vi "ctet_dmm_User Main.vi"() -> ()   [LabVIEW 2019, in "ctet_dmm User Library.lvlib"]
uses:
  ctet_dmm User Library.lvlib
  Servers/ctet_dmm/ctet_dmm Class/typeDefs/Server State Data.ctl
  Types/ctet_dmm.ctl
  Servers/ctet_dmm/ctet_dmm Class/RPC Messages/measurementservice_DMMConfigResponse/measurementservice_DMMConfigResponse_Data.ctl
  Servers/ctet_dmm/ctet_dmm Class/RPC Messages/measurementservice_ErrorOut/measurementservice_ErrorOut_Data.ctl
  Servers/ctet_dmm/ctet_dmm Class/ctet_dmm.lvclass/ctet_dmm.ctl
  Servers/ctet_dmm/ctet_dmm Class/ctet_dmm.lvclass
panel:
  in  "Stop":bool
  in  "Server Address":string="0.0.0.0:50051"
  in  "Server Certificate File (.crt)":path
  in  "Server Key File (.key)":path
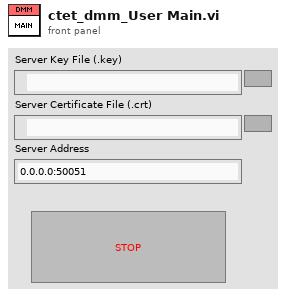
[diagram p1: front panel]
types:
  T1 = typedef "ctet_dmm User Library.lvlib/ctet_dmm.ctl" = cluster{"DMMSession":refnum<k15>, "measurementservice_DMMConfigResponse_Data":T2}
  T2 = typedef "ctet_dmm.lvlib/ctet_dmm.lvclass/measurementservice_DMMConfigResponse_Data.ctl" = cluster{"DMMFunction":i64, "DMMResolution":dbl, "DMMRange":dbl, "DMMSampleCount":i64, "DMMApertureTimeUnit":i64, "DMMApertureTime":dbl, "DMMNumberofAverages":i64, "DMMAutoZero":i64, "DMMADCCalibration":i64, "DMMSettleTime":dbl, "error":T3}
  T3 = typedef "ctet_dmm.lvlib/ctet_dmm.lvclass/measurementservice_ErrorOut_Data.ctl" = cluster{"errCode":i64, "errMessage":string}
  T4 = typedef "ctet_dmm.lvlib/ctet_dmm.lvclass/Server State Data.ctl" = cluster{"Data":string}
  T5 = typedef "ctet_dmm.lvlib/ctet_dmm.lvclass/Server gRPC UEs.ctl" = cluster{"Invoke gRPC UE":refnum<user-event>, "Query gRPC UE":refnum<user-event>, "Register gRPC UE":refnum<user-event>, "OpenDMMSession gRPC UE":refnum<user-event>, "ConfigureDMM gRPC UE":refnum<user-event>, "PerformDMMMeasurement gRPC UE":refnum<user-event>, "CloseDMMSession gRPC UE":refnum<user-event>, "SelfCalibrateDMM gRPC UE":refnum<user-event>, "ResetDMM gRPC UE":refnum<user-event>, "GetDMMLastExtCalInfo gRPC UE":refnum<user-event>, "GetDMMLastSelfCalInfo gRPC UE":refnum<user-event>}
  T6 = typedef "ctet_dmm.lvlib/gprc-lvsupport.lvlib/grpcId.ctl" = u64
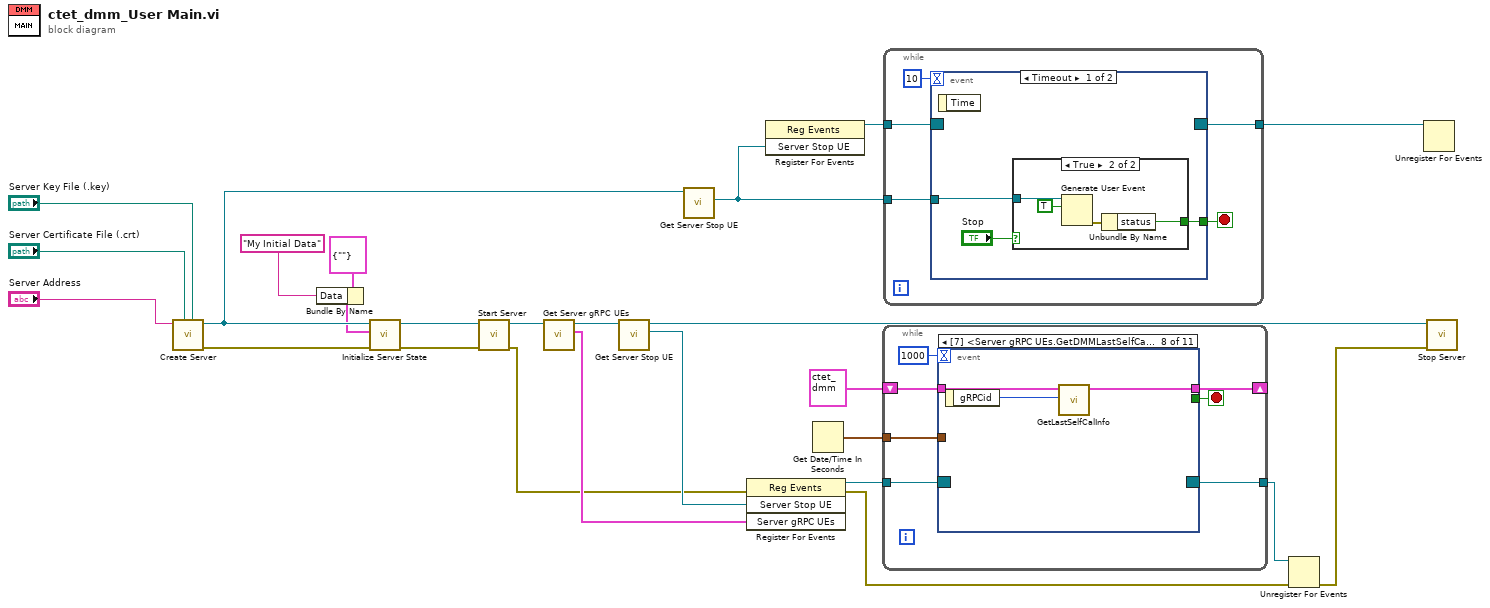
[diagram p0: block diagram]
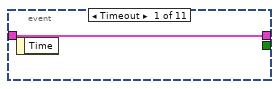
[diagram p2: hidden frame]
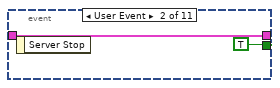
[diagram p3: hidden frame]
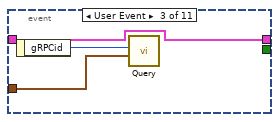
[diagram p4: hidden frame]
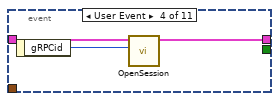
[diagram p5: hidden frame]
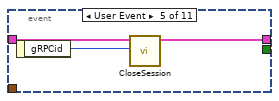
[diagram p6: hidden frame]
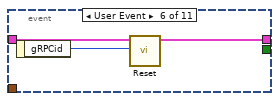
[diagram p7: hidden frame]
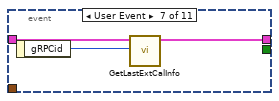
[diagram p8: hidden frame]
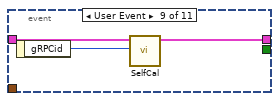
[diagram p9: hidden frame]
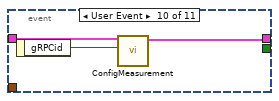
[diagram p10: hidden frame]
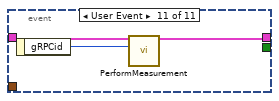
[diagram p11: hidden frame]
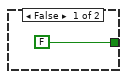
[diagram p12: hidden frame]
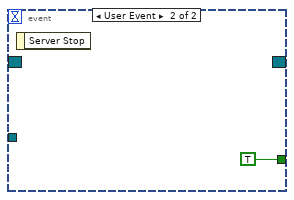
[diagram p13: hidden frame]
diagram:
  n1 = call "Create Server.vi"("Server Key File (.key)"="Server Key File (.key)", "Server Certificate File (.crt)"="Server Certificate File (.crt)", "Server Address"="Server Address") -> ("error out"=w19:errorcluster, "gRPC Server out"=w16:refnum<class "ctet_dmm.lvclass">)  [unwired: 7 in]
  n2 = Bundle By Name(cluster=T4 {"Data"=""} ("Initial State"), "Data"="My Initial Data") -> (w14:T4)
  n3 = call "Initialize Server State.vi"("error in (no error)"=w19, "Initial State"=w14, "gRPC Server in"=w16) -> ("error out"=w18:errorcluster, "gRPC Server out"=w17:refnum<class "ctet_dmm.lvclass">)  [unwired: 7 in]
  n4 = call "Start Server.vi"("error in (no error)"=w18, "gRPC Server in"=w17) -> ("error out"=w6:errorcluster, "gRPC Server out"=w7:refnum<class "ctet_dmm.lvclass">)  [unwired: 8 in]
  n5 = call "Get Server gRPC UEs.vi"("OOP Server in"=w7) -> ("Server gRPC UEs"=w10:T5, "OOP Server out"=w12:refnum<class "ctet_dmm.lvclass">)  [unwired: 9 in]
  n6 = call "Get Server Stop UE.vi"("OOP Server in"=w12) -> ("Server Stop UE"=w11:refnum<user-event>, "OOP Server out"=w3:refnum<class "ctet_dmm.lvclass">)  [unwired: 9 in]
  n7 = call "Get Server Stop UE.vi"("OOP Server in"=w16) -> ("Server Stop UE"=w20:refnum<user-event>)  [unwired: 9 in, 1 out]
  n8 = register-events(error in=w6, w11, w10) -> (reference out=w9:refnum<event-registration>, error out=w5:errorcluster)  [unwired: 1 in]
  n9 = register-events(w20) -> (reference out=w22:refnum<event-registration>)  [unwired: 2 in, 1 out]
  n10 = Get Date/Time In Seconds() -> (seconds since 1Jan1904=w2:timestamp)
  n11 = while {
    tunnel: w9 -> [w32]
    tunnel: [w30] -> w8
    tunnel: w2 -> [w28]
    shift-right: [w26] -> _
    shift-left: T1 {"DMMSession"="", "measurementservice_DMMConfigResponse_Data"={"DMMFunction"=0, "DMMResolution"=0.0, "DMMRange"=0.0, "DMMSampleCount"=0, "DMMApertureTimeUnit"=0, "DMMApertureTime"=0.0, "DMMNumberofAverages"=0, "DMMAutoZero"=0, "DMMADCCalibration"=0, "DMMSettleTime"=0.0, "error"={"errCode"=0, "errMessage"=""}}} ("ctet_dmm") -> [w27]
    stop <- w31 stop-if-true
    n12 = event "RPC Methods Event Structure" shown="[7] <Server gRPC UEs.GetDMMLastSelfCalInfo gRPC UE>: User Event" {
      selector: w32 -> [_ _ _ _ _ _ _ _ _ _ _]
      dyn-events: [_ _ _ _ _ _ _ _ _ _ _] -> w30
      timeout: 1000 -> [_ _ _ _ _ _ _ _ _ _ _]
      tunnel: [_ TRUE _ _ _ _ _ _ _ _ _] -> w31
      tunnel: w28 -> [_ _ w37 _ _ _ _ _ _ _ _]
      tunnel: w27 -> [w33 w34 w36 w40 w44 w47 w50 w53 w56 w59 w62]
      tunnel: [w33 w34 w36 w39 w42 w45 w48 w51 w54 w57 w60] -> w26
      event Timeout {
        n13 = event-data() -> ()  [unwired: 1 in, 1 out]
      }
      event User Event {
        n14 = event-data() -> ()  [unwired: 1 in, 1 out]
      }
      event User Event {
        n15 = event-data() -> ("gRPCid"=w38:T6)  [unwired: 1 in]
        n16 = call "Query.vi"("current time"=w37, "gRPCid"=w38) -> ()  [unwired: 9 in, 1 out]
      }
      event User Event {
        n17 = event-data() -> ("gRPCid"=w41:T6)  [unwired: 1 in]
        n18 = call "OpenSession.vi"("gRPCid"=w41, "ctet_dmm"=w40) -> ("ctet_dmm out"=w39:T1)  [unwired: 8 in, 1 out]
      }
      event User Event {
        n19 = event-data() -> ("gRPCid"=w43:T6)  [unwired: 1 in]
        n20 = call "CloseSession.vi"("gRPCid"=w43, "ctet_dmm"=w44) -> ("ctet_dmm out"=w42:T1)  [unwired: 8 in, 1 out]
      }
      event User Event {
        n21 = event-data() -> ("gRPCid"=w46:T6)  [unwired: 1 in]
        n22 = call "Reset.vi"("gRPCid"=w46, "ctet_dmm"=w47) -> ("ctet_dmm out"=w45:T1)  [unwired: 8 in, 1 out]
      }
      event User Event {
        n23 = event-data() -> ("gRPCid"=w49:T6)  [unwired: 1 in]
        n24 = call "GetLastExtCalInfo.vi"("gRPCid"=w49, "ctet_dmm"=w50) -> ("ctet_dmm out"=w48:T1)  [unwired: 8 in, 1 out]
      }
      event User Event {
        n25 = event-data() -> ("gRPCid"=w52:T6)  [unwired: 1 in]
        n26 = call "GetLastSelfCalInfo.vi"("gRPCid"=w52, "ctet_dmm"=w53) -> ("ctet_dmm out"=w51:T1)  [unwired: 8 in, 1 out]
      }
      event User Event {
        n27 = event-data() -> ("gRPCid"=w55:T6)  [unwired: 1 in]
        n28 = call "SelfCal.vi"("gRPCid"=w55, "ctet_dmm"=w56) -> ("ctet_dmm out"=w54:T1)  [unwired: 8 in, 1 out]
      }
      event User Event {
        n29 = event-data() -> ("gRPCid"=w58:T6)  [unwired: 1 in]
        n30 = call "ConfigMeasurement.vi"("gRPCid"=w58, "ctet_dmm"=w59) -> ("ctet_dmm out"=w57:T1)  [unwired: 8 in, 1 out]
      }
      event User Event {
        n31 = event-data() -> ("gRPCid"=w61:T6)  [unwired: 1 in]
        n32 = call "PerformMeasurement.vi"("gRPCid"=w61, "ctet_dmm"=w62) -> ("ctet_dmm out"=w60:T1)  [unwired: 8 in, 1 out]
      }
    }
  }
  n33 = while {
    tunnel: w20 -> [w67]
    tunnel: w22 -> [w66]
    tunnel: [w64] -> w21
    stop <- w65 stop-if-true
    n34 = event shown="[0] Timeout" {
      selector: w66 -> [_ _]
      dyn-events: [_ _] -> w64
      timeout: 10 -> [_ _]
      tunnel: w67 -> [w70 _]
      tunnel: [w69 TRUE] -> w65
      event Timeout {
        n35 = event-data() -> ()  [unwired: 1 in, 1 out]
        n36 = case shown="True" "Stop" {
          tunnel: w70 -> [_ w73]
          tunnel: [FALSE ("status") w72] -> w69
          frame False {
          }
          frame True {
            n37 = Generate User Event(user event=w73, event data cluster=TRUE ("event data")) -> (error out=w74:errorcluster)  [unwired: 2 in, 1 out]
            n38 = Unbundle By Name(w74) -> ("status"=w72:bool)
          }
        }
      }
      event User Event {
        n39 = event-data() -> ()  [unwired: 1 in, 1 out]
      }
    }
  }
  n40 = Unregister For Events(event registration refnum=w8, error in=w5) -> (error out=w4:errorcluster)
  n41 = Unregister For Events(event registration refnum=w21) -> ()  [unwired: 1 in, 1 out]
  n42 = call "Stop Server.vi"("error in (no error)"=w4, "gRPC Server in"=w3) -> ()  [unwired: 9 in, 1 out]
